vi "12.3 SegementProcess.vi"() -> ()   [LabVIEW 2016]
doc: "This example shows how to use the Edge Tool in NI Vision. The Edge Tool finds edges (or sharp transitions in the pixels values) along a given line or ROI profile. The Edge Tool is a precursor function to many of the gauging and inspection tasks. For example, the location of the edges found along a line profile across an object can interpreted as the boundaries of the object whose dimensions have to be measured for a gauging application or the presence of a crack in the surface of an object for an inspection application."
uses:
  <vilib>/vision/NI_Vision_Development_Module.lvlib
panel:
  in  "Method":T1(ring)
  in  "Tab":T2(tab)
  out "Src":T3(plugin-control)
  out "Bin":T3(plugin-control)
  out "Map":T3(plugin-control)
  out "Bin":T3(plugin-control)
  out "Seg":T3(plugin-control)
  out "Skiz":T3(plugin-control)
  out "Dst":T3(plugin-control)
  in  "Range":cluster{"Lower value":sgl, "Upper value":sgl}={"Lower value"=0.0, "Upper value"=193.0}
  in  "Connectivity":bool=TRUE
  in  "Stop":bool
  # "Instruction:\nRun program, select each method and check out the relevant images and results.\n\nSome Facts:\nFor Labeling, realize only the particles with label from 10-25 were selected;\n\nFor segementation and Skiz, realize they are time comusing and particle can be extracted by their area;\n\nFor watershed, it is fast compare to Skiz and Segementation and the particle can be extracted by seperated by area."
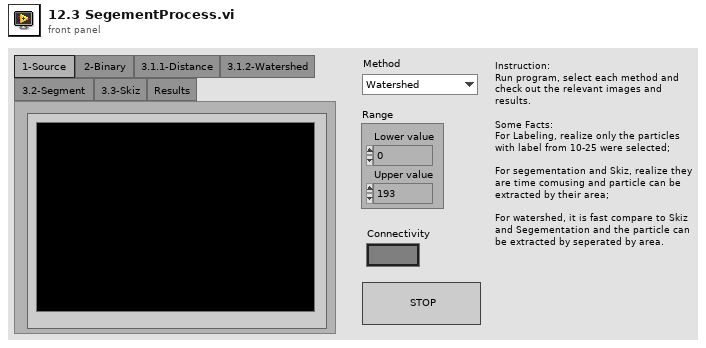
[diagram p1: front panel]
types:
  T1 = enum16{"Watershed", "Labeling", "Segementation", "Skiz"}
  T2 = enum32{"1-Source ", "2-Binary ", "3.1.1-Distance", "3.1.2-Watershed", "3.2-Segment ", "3.3-Skiz", "Results"}
  T3 = typedef "IMAQ Image.ctl" = refnum<image>
  T4 = cluster{"Method":enum16{"Watershed", "Labeling", "Segementation", "Skiz"}, "Range":cluster{"Lower value":sgl, "Upper value":sgl}, "Connectivity":bool}
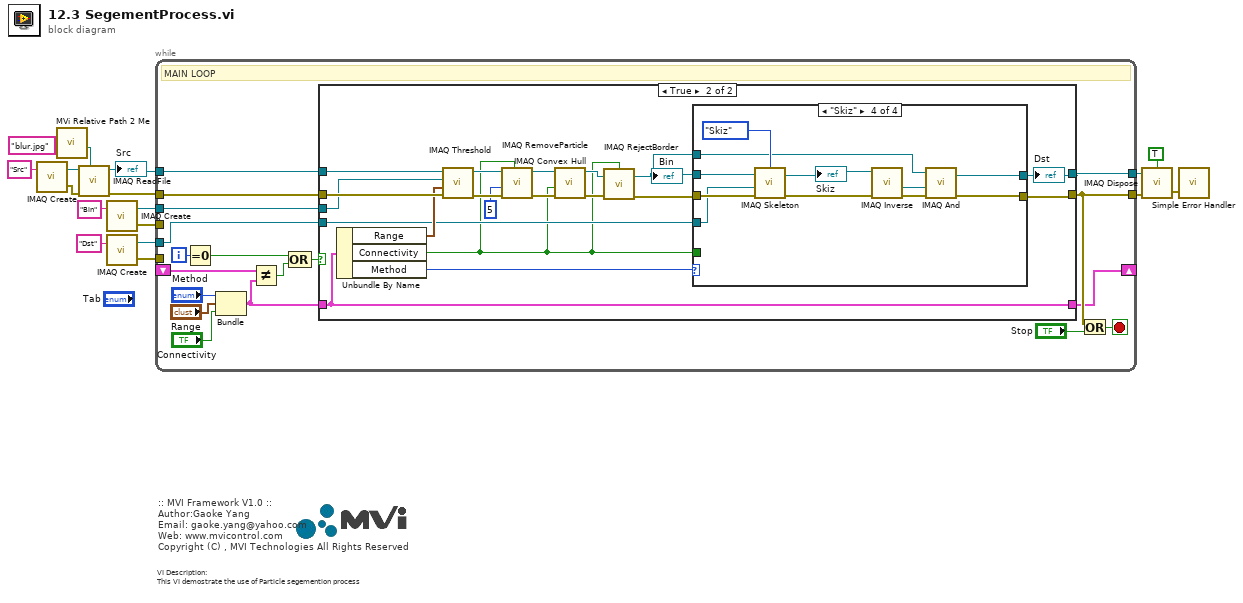
[diagram p0: block diagram]
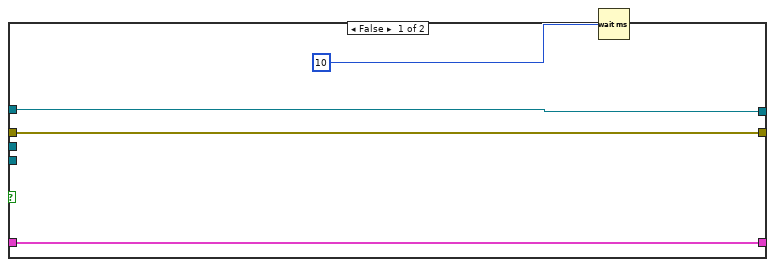
[diagram p2: hidden frame]
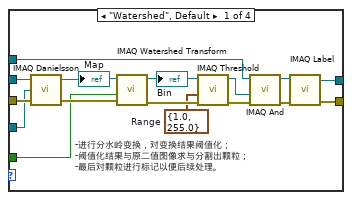
[diagram p3: hidden frame]
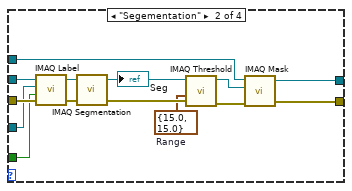
[diagram p4: hidden frame]
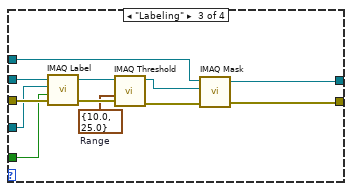
[diagram p5: hidden frame]
diagram:
  # "VI Description:\nThis VI demostrate the use of Particle segemention process"
  # ":: MVI Framework V1.0 ::\nAuthor:Gaoke Yang\nEmail: gaoke.yang@yahoo.com\nWeb: www.mvicontrol.com\nCopyright (C) , MVI Technologies All Rights Reserved"
  n1 = call "IMAQ Create"("Image Name"="Src") -> ("New Image"=w16:T3, "error out"=w15:errorcluster)  [unwired: 4 in]
  n2 = call "MVi Relative Path 2 Me.vi"("Relative Path"="blur.jpg" ("name or relative path")) -> ("Appended Dir"=w11:path)  [unwired: 5 in, 1 out]
  n3 = call "IMAQ ReadFile"("File Path"=w11, "error in (no error)"=w15, "Image"=w16) -> ("error out"=w5:errorcluster, "Image Out"=w4:T3)  [unwired: 4 in, 3 out]
  "Src" <- w4
  n4 = call "IMAQ Create"("Image Name"="Bin") -> ("New Image"=w8:T3, "error out"=w7:errorcluster)  [unwired: 4 in]
  n5 = call "IMAQ Create"("Image Name"="Dst") -> ("New Image"=w2:T3, "error out"=w1:errorcluster)  [unwired: 4 in]
  n6 = while "MAIN LOOP" {
    tunnel: w4 -> [w34]
    tunnel: w5 -> [w35]
    tunnel: [w30] -> w14
    tunnel: [w31] -> w13
    shift-right: [w27] -> _
    shift-left: _ -> [w25]
    tunnel: w8 -> [w23]
    tunnel: w7 -> [_]
    tunnel: w2 -> [w18]
    tunnel: w1 -> [_]
    i -> [w29]
    stop <- w32 stop-if-true
    # "MAIN LOOP"
    n7 = Equal To 0?(x=w29) -> (x = 0?=w26:bool)
    n8 = Bundle("Method"="Method", "Range"="Range", "Connectivity"="Connectivity") -> (w22:T4)  [unwired: 1 in]
    n9 = Not Equal?(x=w25, y=w22) -> (x != y?=w24:bool)
    n10 = Compound Arithmetic op=OR(w26, w24) -> (w28:bool)
    n11 = case shown="True" w28 {
      tunnel: w35 -> [w38 w58]
      tunnel: w34 -> [w39 w57]
      tunnel: [w39 w52] -> w31
      tunnel: [w38 w53] -> w30
      tunnel: [w36 w56] -> w27
      tunnel: w22 -> [w36 w56]
      tunnel: w23 -> [_ w51]
      tunnel: w18 -> [_ w50]
      frame False {
        n12 = Wait (ms)(milliseconds to wait=u32 10) -> ()  [unwired: 1 out]
      }
      frame True {
        n13 = Unbundle By Name(w56) -> ("Range"=w55:cluster{"Lower value":sgl, "Upper value":sgl}, "Connectivity"=w40:bool, "Method"=w54:T1)
        n14 = call "IMAQ Threshold"("error in (no error)"=w58, "Range"=w55, "Image Dst"=w51, "Image Src"=w57) -> ("error out"=w45:errorcluster, "Image Dst Out"=w44:T3)  [unwired: 6 in]
        n15 = call "IMAQ RemoveParticle"("Connectivity 4/8 (8)"=w40, "error in (no error)"=w45, "Number of Erosion"=5, "Image Src"=w44) -> ("error out"=w43:errorcluster, "Image Dst Out"=w42:T3)  [unwired: 6 in]
        n16 = call "IMAQ Convex Hull"("error in (no error)"=w43, "Connectivity 4/8 (8)"=w40, "Image Src"=w42) -> ("error out"=w49:errorcluster, "Image Dst Out"=w48:T3)  [unwired: 7 in]
        n17 = call "IMAQ RejectBorder"("error in (no error)"=w49, "Image Src"=w48, "Connectivity 4/8 (8)"=w40) -> ("error out"=w47:errorcluster, "Image Dst Out"=w46:T3)  [unwired: 3 in]
        "Bin" <- w46
        n18 = case shown="\"Skiz\"" w54 {
          tunnel: w47 -> [w74 w88 w100 w111]
          tunnel: w46 -> [w73 w87 w99 w110]
          tunnel: w40 -> [w71 w85 w89 _]
          tunnel: w46 -> [w66 w76 w94 w104]
          tunnel: w50 -> [w65 w86 w95 w109]
          tunnel: [w62 w80 w92 w105] -> w53
          tunnel: [w61 w79 w90 w103] -> w52
          frame "Watershed", Default {
            w63 = cluster{"Lower value":sgl, "Upper value":sgl} {"Lower value"=1.0, "Upper value"=255.0}  # Range
            # "-进行分水岭变换，对变换结果阈值化；\n-阈值化结果与原二值图像求与分割出颗粒；\n-最后对颗粒进行标记以便后续处理。"
            n19 = call "IMAQ Danielsson"("error in (no error)"=w74, "Image Dst"=w65, "Image Src"=w73) -> ("error out"=w72:errorcluster, "Image Dst Out"=w59:T3)  [unwired: 1 in]
            "Map" <- w59
            n20 = call "IMAQ Watershed Transform"("error in (no error)"=w72, "Connectivity 4/8 (8)"=w71, "Image Src"=w59) -> ("error out"=w67:errorcluster, "Image Dst Out"=w60:T3)  [unwired: 6 in, 1 out]
            "Bin" <- w60
            n21 = call "IMAQ Threshold"("error in (no error)"=w67, "Range"=w63, "Image Src"=w60) -> ("error out"=w68:errorcluster, "Image Dst Out"=w64:T3)  [unwired: 3 in, 4 out]
            n22 = call "IMAQ And"("error in (no error)"=w68, "Image Src B"=w64, "Image Src A"=w66) -> ("error out"=w70:errorcluster, "Image Dst Out"=w69:T3)  [unwired: 7 in]
            n23 = call "IMAQ Label"("error in (no error)"=w70, "Image Src"=w69) -> ("error out"=w62:errorcluster, "Image Dst Out"=w61:T3)  [unwired: 2 in, 1 out]
          }
          frame "Segementation" {
            w78 = cluster{"Lower value":sgl, "Upper value":sgl} {"Lower value"=15.0, "Upper value"=15.0}  # Range
            n24 = call "IMAQ Label"("error in (no error)"=w88, "Connectivity 4/8 (8)"=w85, "Image Dst"=w86, "Image Src"=w87) -> ("error out"=w84:errorcluster, "Image Dst Out"=w83:T3)  [unwired: 1 out]
            n25 = call "IMAQ Segmentation"("error in (no error)"=w84, "Image Src"=w83) -> ("error out"=w82:errorcluster, "Image Dst Out"=w75:T3)  [unwired: 2 in]
            "Seg" <- w75
            n26 = call "IMAQ Threshold"("error in (no error)"=w82, "Range"=w78, "Image Src"=w75) -> ("error out"=w81:errorcluster, "Image Dst Out"=w77:T3)  [unwired: 3 in, 4 out]
            n27 = call "IMAQ Mask"("error in (no error)"=w81, "Image Mask"=w77, "Image Src"=w76) -> ("error out"=w80:errorcluster, "Image Dst Out"=w79:T3)  [unwired: 2 in]
          }
          frame "Labeling" {
            w97 = cluster{"Lower value":sgl, "Upper value":sgl} {"Lower value"=10.0, "Upper value"=25.0}  # Range
            n28 = call "IMAQ Label"("error in (no error)"=w100, "Connectivity 4/8 (8)"=w89, "Image Dst"=w95, "Image Src"=w99) -> ("error out"=w98:errorcluster, "Image Dst Out"=w91:T3)  [unwired: 1 out]
            n29 = call "IMAQ Threshold"("error in (no error)"=w98, "Range"=w97, "Image Src"=w91) -> ("error out"=w96:errorcluster, "Image Dst Out"=w93:T3)  [unwired: 3 in, 4 out]
            n30 = call "IMAQ Mask"("error in (no error)"=w96, "Image Mask"=w93, "Image Src"=w94) -> ("error out"=w92:errorcluster, "Image Dst Out"=w90:T3)  [unwired: 2 in]
          }
          frame "Skiz" {
            n31 = call "IMAQ Skeleton"("error in (no error)"=w111, "Image Dst"=w109, "Image Src"=w110, "Mode"=enum32{"Skeleton L", "Skeleton M", "Skiz"}."Skiz") -> ("error out"=w107:errorcluster, "Image Dst Out"=w101:T3)  [unwired: 2 in]
            "Skiz" <- w101
            n32 = call "IMAQ Inverse"("error in (no error)"=w107, "Image Src"=w101) -> ("error out"=w106:errorcluster, "Image Dst Out"=w102:T3)  [unwired: 8 in]
            n33 = call "IMAQ And"("error in (no error)"=w106, "Image Src B"=w102, "Image Src A"=w104) -> ("error out"=w105:errorcluster, "Image Dst Out"=w103:T3)  [unwired: 7 in]
          }
        }
        "Dst" <- w52
      }
    }
    n34 = Or(x=w30, y="Stop") -> (x .or. y?=w32:bool)
  }
  n35 = call "IMAQ Dispose"("All Images? (No)"=TRUE, "Image"=w13, "error in (no error)"=w14) -> ("error out"=w10:errorcluster)  [unwired: 3 in]
  n36 = call <vilib>:"Simple Error Handler.vi"("error in (no error)"=w10) -> ()  [unwired: 4 in, 5 out]
